vi "Talon_Limit_Switch.vi"() -> ()   [LabVIEW 2012]
uses:
  <vilib>/Rock Robotics/WPI/DigitalInput/WPI_DigitalInputDevRef.ctl
  <vilib>/Rock Robotics/SystemInterfaces/DIO/FPGA_DIOChannel.ctl
  <vilib>/Rock Robotics/SystemInterfaces/Typedef/FPGA_TypedefDigitalModule.ctl
  <vilib>/Rock Robotics/SystemInterfaces/DIO/FPGA_DIOPWMChannel.ctl
  <vilib>/Rock Robotics/WPI/Joystick/WPI_JoystickAxis.ctl
  <vilib>/Rock Robotics/WPI/MotorControl/WPI_MotorControlOpen Talon.vi
  <vilib>/Rock Robotics/WPI/Joystick/WPI_JoystickGetSetRefNum.vi
panel:
  in  "Launcher":T1
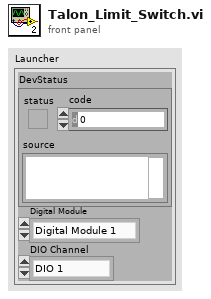
[diagram p1: front panel]
types:
  T1 = typedef "WPI_DigitalInputDevRef.ctl" = cluster{"DevStatus":errorcluster, "DIO Channel":T2, "Digital Module":T3}
  T2 = typedef "FPGA_DIOChannel.ctl" = enum8{"DIO 1", "DIO 2", "DIO 3", "DIO 4", "DIO 5", "DIO 6", "DIO 7", "DIO 8", "DIO 9", "DIO 10", "DIO 11", "DIO 12", "DIO 13", "DIO 14", "Invalid"}
  T3 = typedef "FPGA_TypedefDigitalModule.ctl" = enum16{"Digital Module 1", "Digital Module 2"}
  T4 = typedef "FPGA_DIOPWMChannel.ctl" = enum8{"PWM 1", "PWM 2", "PWM 3", "PWM 4", "PWM 5", "PWM 6", "PWM 7", "PWM 8", "PWM 9", "PWM 10", "Invalid"}
  T5 = typedef "WPI_MotorControlDeviceRef.ctl" = cluster{"DeviceStatus":errorcluster, "Type":enum16{"PWM", "CAN"}, "PWM":cluster{"Digital Module":T3, "PWM Channel":T4, "DeadBand":T6}, "CAN":cluster{"Device Number":u8, "Control Mode":T7, "Semaphore":T8, "Max Vout":dbl}, "Invert":bool, "TransformRef":T9, "InvTransformRef":T9}
  T6 = typedef "WPI_PWMDeadband.ctl" = cluster{"Name":string, "maxPositivePwm":i32, "minPositivePwm":i32, "centerPwm":i32, "maxNegativePwm":i32, "minNegativePwm":i32, "angularRange":u16}
  T7 = typedef "WPI_CANJaguar_ControlMode.ctl" = enum8{"Percent VBus", "Current", "Speed", "Position", "Voltage"}
  T8 = typedef "Semaphore RefNum" = refnum<k1>
  T9 = typedef "WPI_PWMTransform_ConPane.ctl" = refnum<vi>
  T10 = typedef "WPI_JoystickDevRef.ctl" = cluster{"Device":T11}
  T11 = typedef "WPI_JoystickDeviceEnum.ctl" = enum16{"USB 1", "USB 2", "USB 3", "USB 4", "Kinect 1", "Kinect 2"}
  T12 = typedef "WPI_JoystickAxis.ctl" = enum16{"Axis 1", "Axis 2", "Axis 3", "Axis 4", "Axis 5", "Axis 6"}
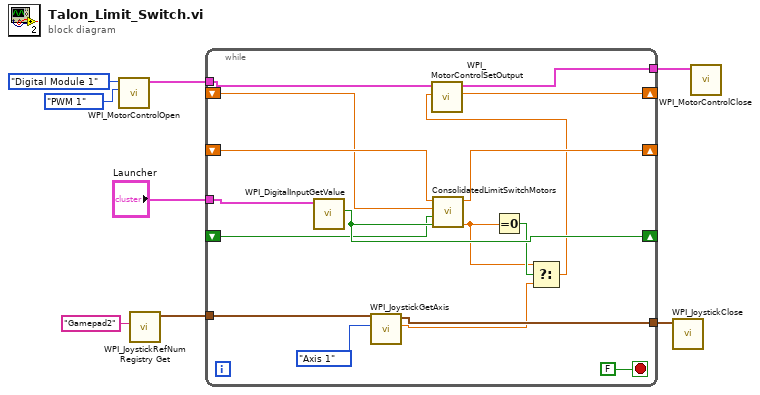
[diagram p0: block diagram]
diagram:
  n1 = call-poly <vilib>:"WPI_MotorControlOpen.vi"("PWM Channel"=FPGA_DIOPWMChannel."PWM 1", "Digital Module (Module 1)"=FPGA_TypedefDigitalModule."Digital Module 1") -> ("MotorControlDeviceRef"=w5:T5)  [unwired: 8 in, 1 out]
  n2 = call <vilib>:"WPI_JoystickRefNum Registry Get.vi"("refnum name"="Gamepad2") -> ("JoystickDevRef"=w4:T10)  [unwired: 9 in, 1 out]
  n3 = while {
    tunnel: w5 -> [w25]
    tunnel: w4 -> [w22]
    tunnel: [w24] -> w3
    shift-right: [w19] -> _
    shift-left: _ -> [w13]
    tunnel: [w20] -> w2
    shift-right: [w17] -> _
    shift-left: _ -> [w16]
    tunnel: "Launcher" -> [w18]
    shift-right: [w15] -> _
    shift-left: _ -> [w14]
    stop <- FALSE stop-if-true
    n4 = call <vilib>:"WPI_DigitalInputGetValue.vi"("DigitalInputDevRef"=w18) -> ("Value"=w17:bool)  [unwired: 8 in, 2 out]
    n5 = call <vilib>:"WPI_JoystickGetAxis.vi"("Axis"=WPI_JoystickAxis."Axis 1", "JoystickDevRef"=w22) -> ("Value"=w9:dbl, "JoystickDevRef"=w20:T10)  [unwired: 8 in]
    n6 = call "ConsolidatedLimitSwitchMotors.vi"("CurrentLSValue"=w17, "LastLSValue"=w16, "CurrentInput"=w13, "LastSign"=w14) -> ("New Output"=w10:dbl, "NewSign"=w15:dbl)  [unwired: 6 in]
    n7 = Equal To 0?(x=w10) -> (x = 0?=w12:bool)
    n8 = Select(t=w10, s=w12, f=w9) -> (s? t:f=w11:dbl)
    n9 = call <vilib>:"WPI_MotorControlSetOutput.vi"("Output"=w11, "MotorControlDevRef"=w25) -> ("Motor Output"=w19:dbl, "MotorControlDevRef"=w24:T5)  [unwired: 7 in, 1 out]
  }
  n10 = call <vilib>:"WPI_JoystickClose.vi"("JoystickDevRef"=w2) -> ()  [unwired: 11 in]
  n11 = call <vilib>:"WPI_MotorControlClose.vi"("MotorControlDevRef"=w3) -> ()  [unwired: 10 in, 1 out]
